vi "loadHTOutcount.vi"() -> ()   [LabVIEW 2012]
uses:
  <vilib>/Utility/file.llb/Read From Spreadsheet File (string).vi
panel:
  out "output cluster 2":T1
  in  "input cluster 2":T1
  out "before substring 5":string
  out "before substring 4":string
  in  "path":path=path "C:/temp/ht"
  out "filenames":string[](array[string])
  out "time stamp":timestamp
  out "SQLDateTime":string
  out "output cluster":T2
  in  "input cluster":T2
  out "all rows":string[][](array[string])
  out "size(s)":i32[](array[numeric])
  in  "file path (dialog if empty)":path=path "C:/temp/ht/G04N19.1S-1_09_07_00.txt"
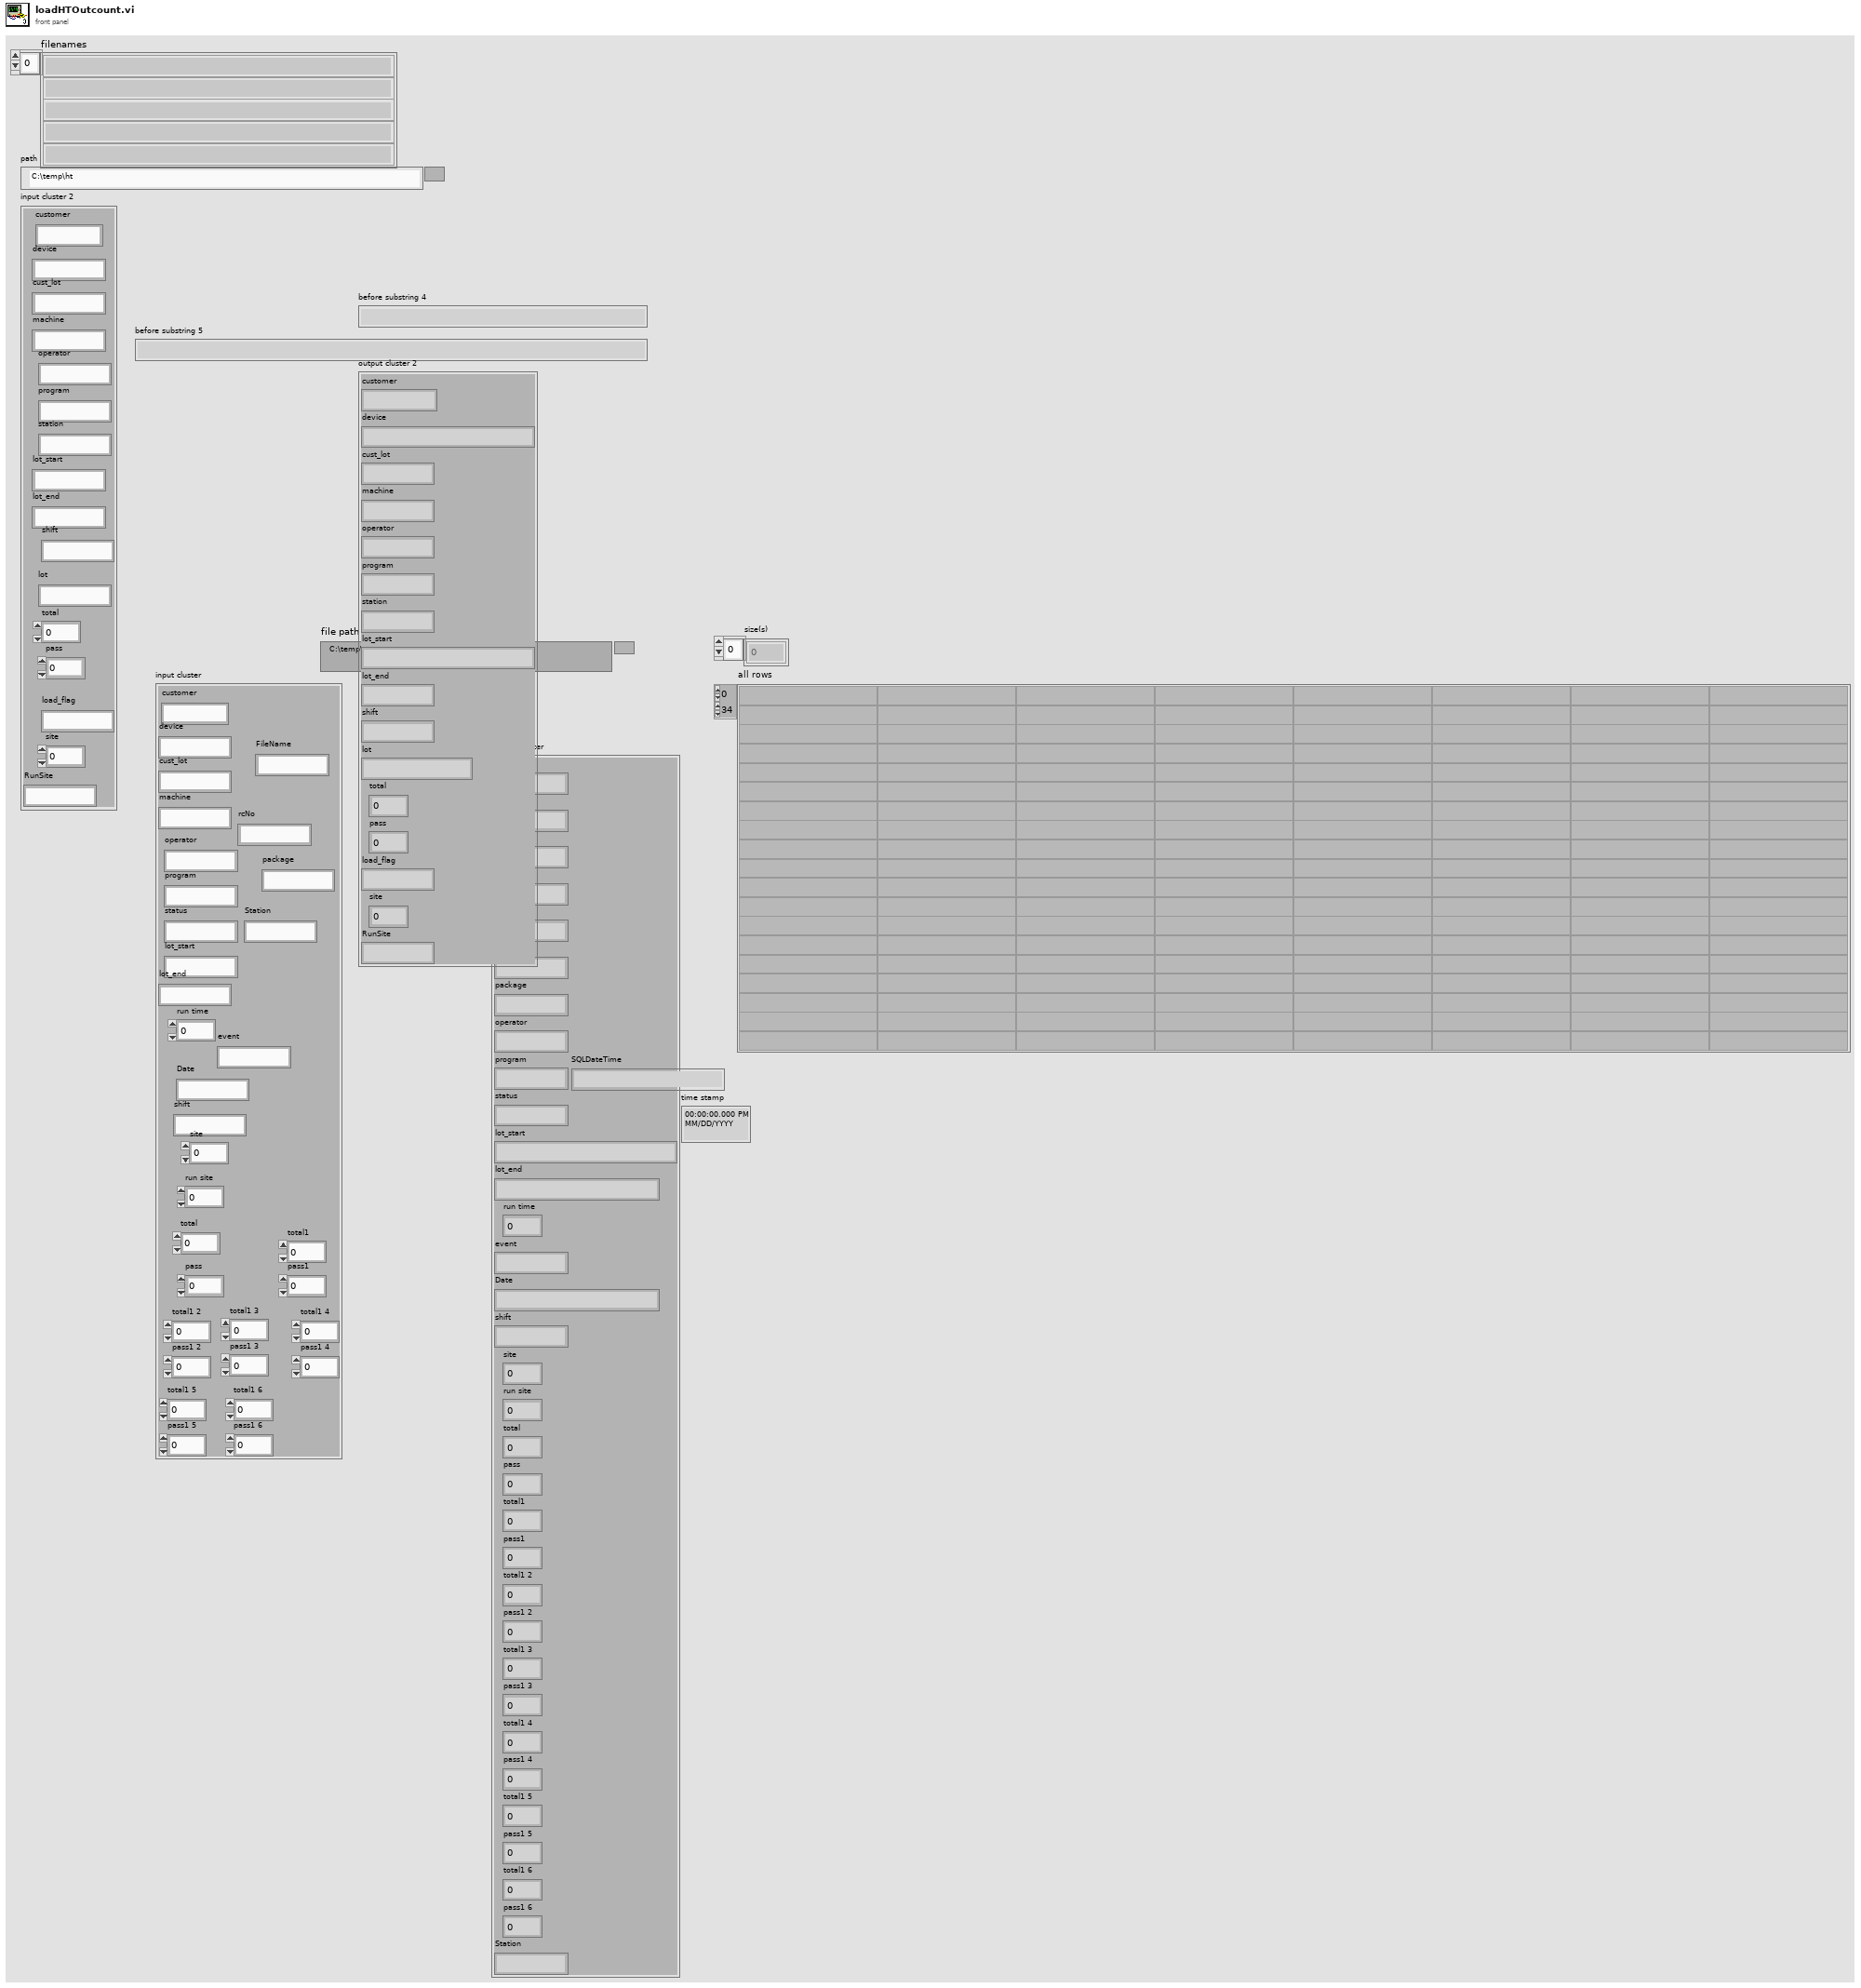
[diagram p1: front panel]
types:
  T1 = cluster{"customer":string, "device":string, "cust_lot":string, "machine":string, "operator":string, "program":string, "station":string, "lot_start":string, "lot_end":string, "shift":string, "lot":string, "total":dbl, "pass":dbl, "load_flag":string, "site":dbl, "RunSite":string}
  T2 = cluster{"customer":string, "device":string, "FileName":string, "cust_lot":string, "machine":string, "rcNo":string, "package":string, "operator":string, "program":string, "status":string, "lot_start":string, "lot_end":string, "run time":dbl, "event":string, "Date":string, "shift":string, "site":dbl, "run site ":dbl, "total":dbl, "pass":dbl, "total1":dbl, "pass1":dbl, "total1 2":dbl, "pass1 2":dbl, "total1 3":dbl, "pass1 3":dbl, "total1 4":dbl, "pass1 4":dbl, "total1 5":dbl, "pass1 5":dbl, "total1 6":dbl, "pass1 6":dbl, "Station":string}
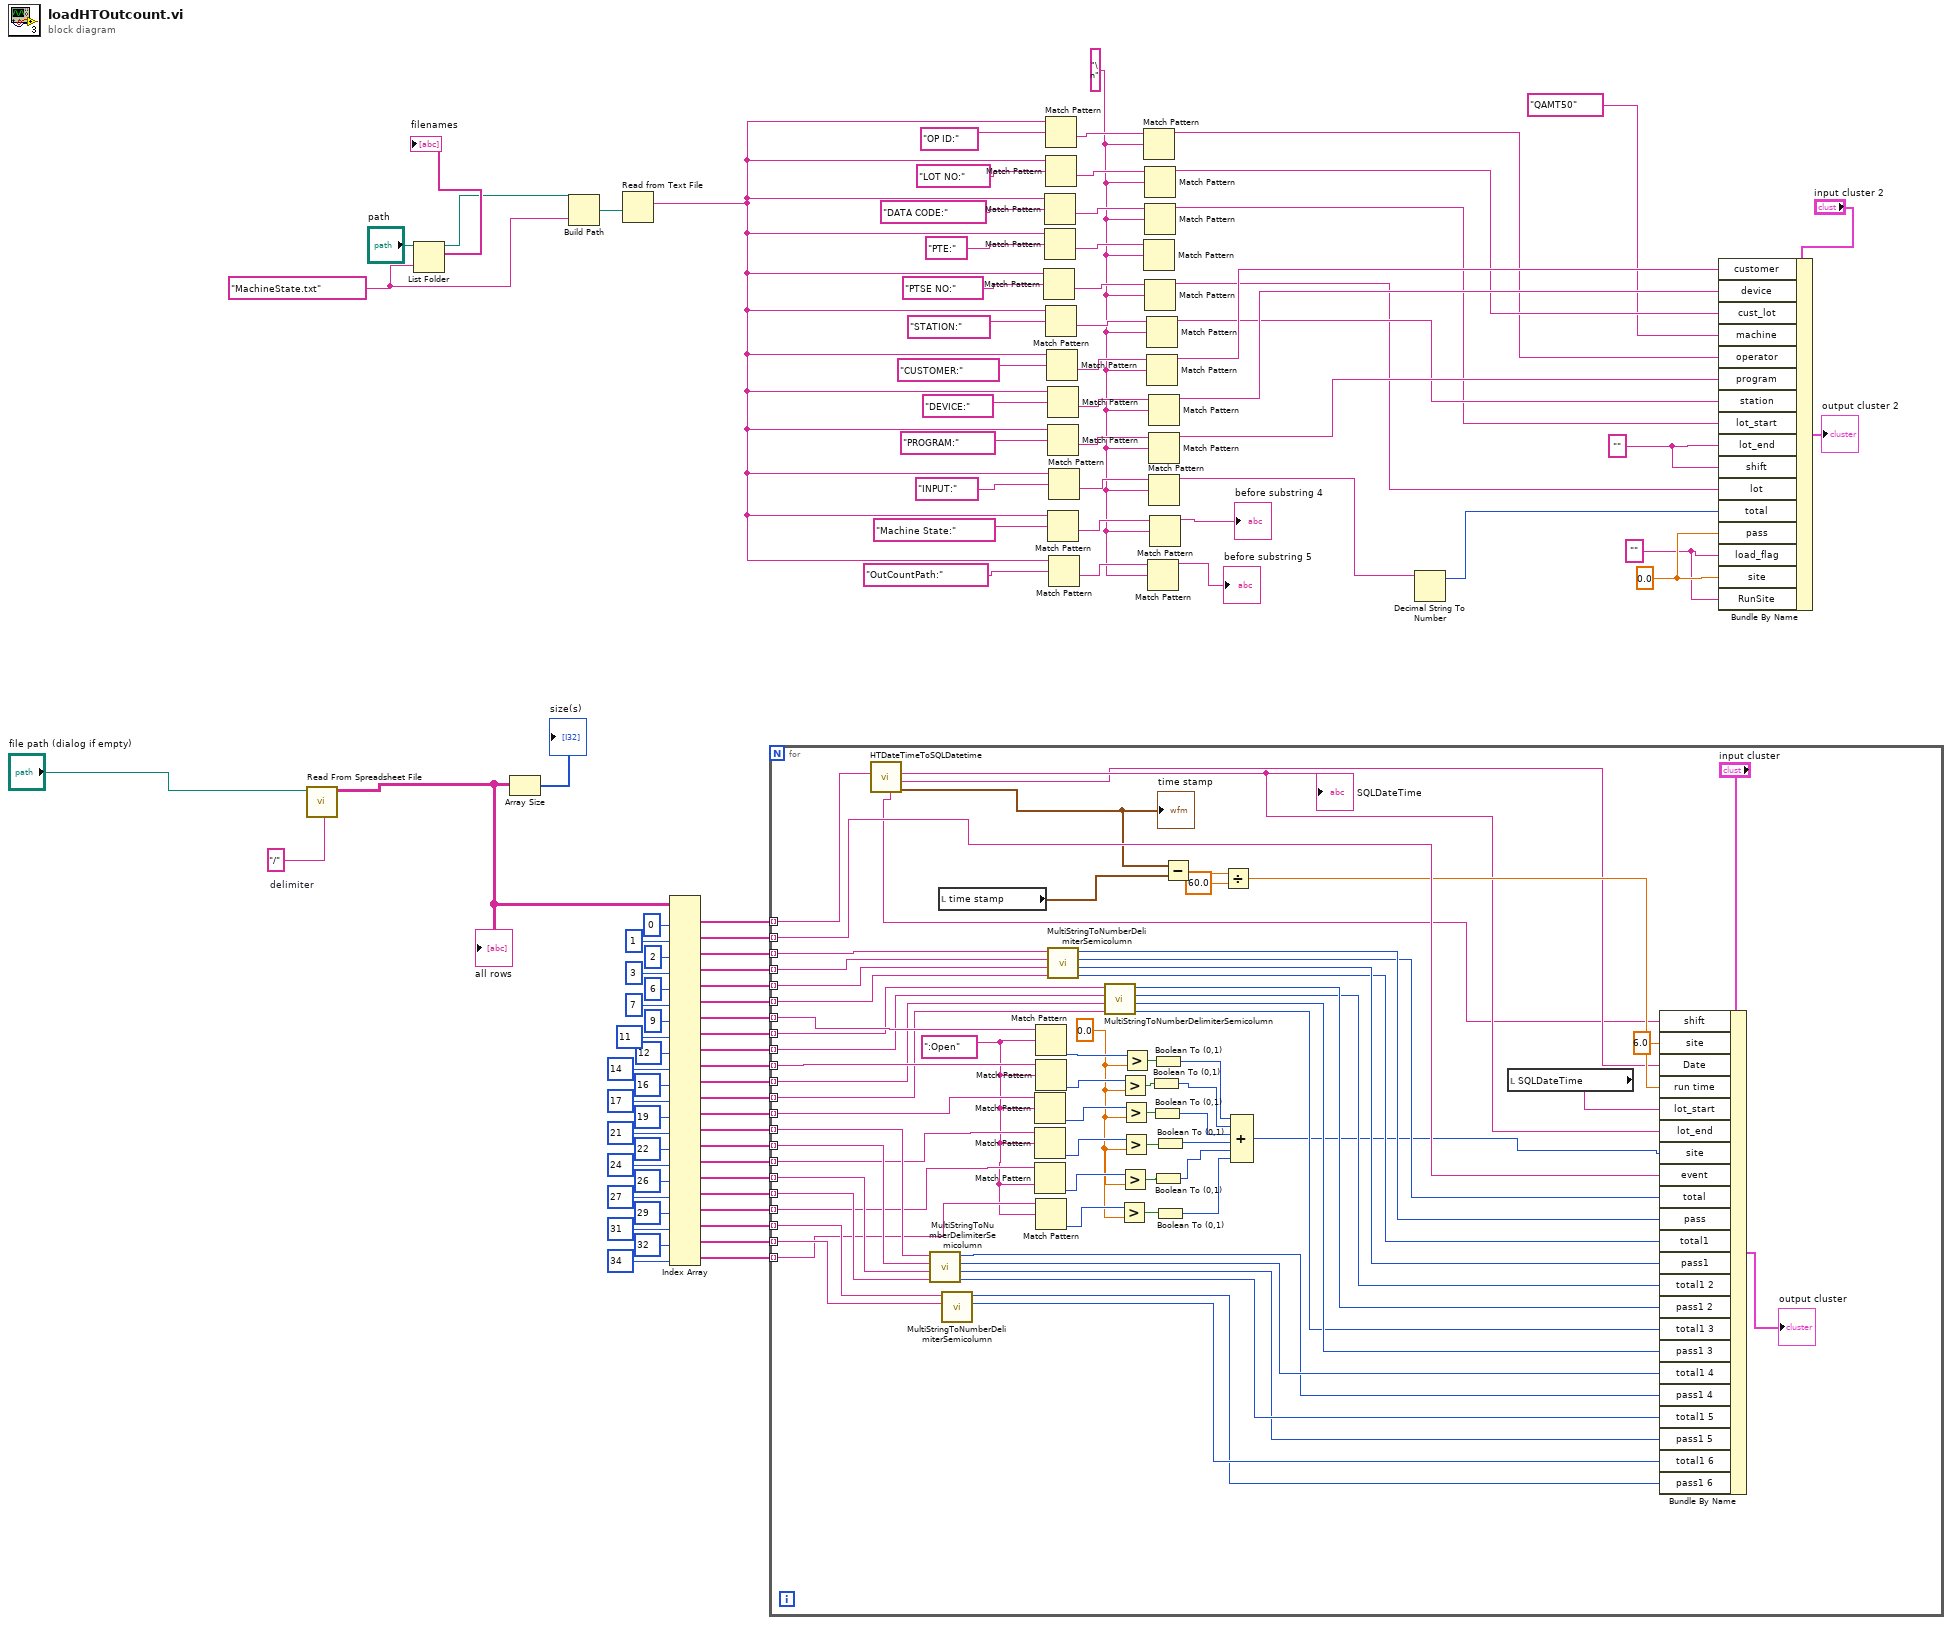
[diagram p0: block diagram]
diagram:
  w3 = "" ("load_flag")
  w4 = 0.0 ("site")
  w7 = "" ("lot_end")
  w1 = "\n" ("regular expression")
  w20 = "MachineState.txt" ("pattern")
  w97 = "/"  # delimiter
  n1 = call-poly <vilib>:"Read From Spreadsheet File.vi"("delimiter (\\t)"=w97, "file path (dialog if empty)"="file path (dialog if empty)") -> ("all rows"=w94:string[][])  [unwired: 5 in, 4 out]
  "all rows" <- w94
  n2 = List Folder(path="path", pattern=w20) -> (path out=w48:path, filenames=→"filenames":string[])  [unwired: 2 in, 2 out]
  n3 = Array Size(array=w94) -> (size(s)=→"size(s)":i32[])
  n4 = Build Path(base path=w48, name or relative path=w20) -> (appended path=w46:path)
  n5 = Read from Text File(file (use dialog)=w46) -> (text=w45:string)  [unwired: 3 in, 3 out]
  n6 = Index Array(array=w94, index (col) #1=0 ("disabled index (col)"), index (col) #2=1 ("index (col)"), index (col) #3=2 ("index (col)"), index (col) #4=3 ("index (col)"), index (col) #5=6 ("index (col)"), index (col) #6=7 ("index (col)"), index (col) #7=9 ("index (col)"), index (col) #8=11 ("index (col)"), index (col) #9=12 ("index (col)"), index (col) #10=14 ("index (col)"), index (col) #11=16 ("index (col)"), index (col) #12=17 ("index (col)"), index (col) #13=19 ("index (col)"), index (col) #14=21 ("index (col)"), index (col) #15=22 ("index (col)"), index (col) #16=24 ("index (col)"), index (col) #17=26 ("index (col)"), index (col) #18=27 ("index (col)"), index (col) #19=29 ("index (col)"), index (col) #20=31 ("index (col)"), index (col) #21=32 ("index (col)"), index (col) #22=34 ("index (col)")) -> (element #1=w92:string[], element #2=w90:string[], element #3=w87:string[], element #4=w86:string[], element #5=w83:string[], element #6=w82:string[], element #7=w80:string[], element #8=w77:string[], element #9=w76:string[], element #10=w74:string[], element #11=w71:string[], element #12=w70:string[], element #13=w68:string[], element #14=w65:string[], element #15=w64:string[], element #16=w62:string[], element #17=w59:string[], element #18=w58:string[], element #19=w56:string[], element #20=w53:string[], element #21=w52:string[], element #22=w50:string[])  [unwired: 22 in]
  n7 = for {
    tunnel: w92 -> [w166] mode=indexing
    tunnel: w90 -> [w130] mode=indexing
    tunnel: w87 -> [w164] mode=indexing
    tunnel: w86 -> [w163] mode=indexing
    tunnel: w83 -> [w162] mode=indexing
    tunnel: w82 -> [w161] mode=indexing
    tunnel: w80 -> [w165] mode=indexing
    tunnel: w77 -> [w160] mode=indexing
    tunnel: w76 -> [w159] mode=indexing
    tunnel: w74 -> [w158] mode=indexing
    tunnel: w71 -> [w157] mode=indexing
    tunnel: w70 -> [w156] mode=indexing
    tunnel: w68 -> [w155] mode=indexing
    tunnel: w65 -> [w154] mode=indexing
    tunnel: w64 -> [w153] mode=indexing
    tunnel: w62 -> [w152] mode=indexing
    tunnel: w59 -> [w151] mode=indexing
    tunnel: w58 -> [w150] mode=indexing
    tunnel: w56 -> [w149] mode=indexing
    tunnel: w53 -> [w148] mode=indexing
    tunnel: w52 -> [w147] mode=indexing
    tunnel: w50 -> [w129] mode=indexing
    w121 = 0.0 ("y")
    w128 = ":Open" ("regular expression")
    n8 = call "HTDateTimeToSQLDatetime.vi"("HTDateTime"=w166) -> ("time stamp"=w105:timestamp, "date string"=w100:string, "SQLDateTime"=w101:string, "Shift"=w98:string)  [unwired: 7 in]
    "SQLDateTime" <- w101
    "time stamp" <- w105
    n9 = call "MultiStringToNumberDelimiterSemicolumn.vi"("input string 4"=w150, "input string 3"=w151, "input string 2"=w153, "input string"=w154) -> ("number 4"=w143:i32, "number 3"=w142:i32, "number 2"=w141:i32, "number"=w140:i32)  [unwired: 4 in]
    n10 = local read "time stamp"() -> (w106:timestamp)
    n11 = call "MultiStringToNumberDelimiterSemicolumn.vi"("input string 2"=w147, "input string"=w148) -> ("number 2"=w145:i32, "number"=w144:i32)  [unwired: 6 in, 2 out]
    n12 = Match Pattern(string=w155, regular expression=w128) -> (offset past match=w125:i32)  [unwired: 1 in, 3 out]
    n13 = Match Pattern(string=w152, regular expression=w128) -> (offset past match=w124:i32)  [unwired: 1 in, 3 out]
    n14 = Match Pattern(string=w149, regular expression=w128) -> (offset past match=w123:i32)  [unwired: 1 in, 3 out]
    n15 = Match Pattern(string=w165, regular expression=w128) -> (offset past match=w127:i32)  [unwired: 1 in, 3 out]
    n16 = Match Pattern(string=w158, regular expression=w128) -> (offset past match=w126:i32)  [unwired: 1 in, 3 out]
    n17 = Match Pattern(string=w129, regular expression=w128) -> (offset past match=w122:i32)  [unwired: 1 in, 3 out]
    n18 = call "MultiStringToNumberDelimiterSemicolumn.vi"("input string 4"=w161, "input string 3"=w162, "input string 2"=w163, "input string"=w164) -> ("number 4"=w134:i32, "number 3"=w135:i32, "number 2"=w132:i32, "number"=w133:i32)  [unwired: 4 in]
    n19 = call "MultiStringToNumberDelimiterSemicolumn.vi"("input string 4"=w156, "input string 3"=w157, "input string 2"=w159, "input string"=w160) -> ("number 4"=w138:i32, "number 3"=w139:i32, "number 2"=w136:i32, "number"=w137:i32)  [unwired: 4 in]
    n20 = Greater?(x=w122, y=w121) -> (0:w117:bool)
    n21 = Greater?(x=w126, y=w121) -> (0:w119:bool)
    n22 = Greater?(x=w123, y=w121) -> (0:w115:bool)
    n23 = Greater?(x=w125, y=w121) -> (0:w116:bool)
    n24 = Greater?(x=w124, y=w121) -> (0:w118:bool)
    n25 = Greater?(x=w127, y=w121) -> (0:w120:bool)
    n26 = Boolean To (0,1)(Boolean=w119) -> (0, 1=w113:i16)
    n27 = Boolean To (0,1)(Boolean=w116) -> (0, 1=w112:i16)
    n28 = Boolean To (0,1)(Boolean=w120) -> (0, 1=w114:i16)
    n29 = Boolean To (0,1)(Boolean=w115) -> (0, 1=w110:i16)
    n30 = Boolean To (0,1)(Boolean=w118) -> (0, 1=w111:i16)
    n31 = Boolean To (0,1)(Boolean=w117) -> (0, 1=w109:i16)
    n32 = Subtract(x=w105, y=w106) -> (x-y=w104:dbl)
    n33 = Divide(x=w104, y=60.0) -> (x/y=w102:dbl)
    n34 = Compound Arithmetic op=ADD(w114, w113, w112, w111, w110, w109) -> (w108:i16)
    n35 = local read "SQLDateTime"() -> (w107:string)
    n36 = Bundle By Name(cluster="input cluster", "shift"=w98, "site"=6.0, "Date"=w100, "run time"=w102, "lot_start"=w107, "lot_end"=w101, "site"=w108, "event"=w130, "total"=w132, "pass"=w133, "total1"=w134, "pass1"=w135, "total1 2"=w136, "pass1 2"=w137, "total1 3"=w138, "pass1 3"=w139, "total1 4"=w141, "pass1 4"=w140, "total1 5"=w143, "pass1 5"=w142, "total1 6"=w145, "pass1 6"=w144) -> (→"output cluster":T2)
  }
  n37 = Match Pattern(string=w45, regular expression="PTSE NO:") -> (after substring=w35:string)  [unwired: 1 in, 3 out]
  n38 = Match Pattern(string=w45, regular expression="DATA CODE:") -> (after substring=w39:string)  [unwired: 1 in, 3 out]
  n39 = Match Pattern(string=w45, regular expression="PTE:") -> (after substring=w37:string)  [unwired: 1 in, 3 out]
  n40 = Match Pattern(string=w45, regular expression="OP ID:") -> (after substring=w43:string)  [unwired: 1 in, 3 out]
  n41 = Match Pattern(string=w45, regular expression="LOT NO:") -> (after substring=w41:string)  [unwired: 1 in, 3 out]
  n42 = Match Pattern(string=w45, regular expression="STATION:") -> (after substring=w22:string)  [unwired: 1 in, 3 out]
  n43 = Match Pattern(string=w45, regular expression="CUSTOMER:") -> (after substring=w33:string)  [unwired: 1 in, 3 out]
  n44 = Match Pattern(string=w45, regular expression="DEVICE:") -> (after substring=w31:string)  [unwired: 1 in, 3 out]
  n45 = Match Pattern(string=w45, regular expression="PROGRAM:") -> (after substring=w29:string)  [unwired: 1 in, 3 out]
  n46 = Match Pattern(string=w45, regular expression="Machine State:") -> (after substring=w25:string)  [unwired: 1 in, 3 out]
  n47 = Match Pattern(string=w45, regular expression="INPUT:") -> (after substring=w27:string)  [unwired: 1 in, 3 out]
  n48 = Match Pattern(string=w45, regular expression="OutCountPath:") -> (after substring=w23:string)  [unwired: 1 in, 3 out]
  n49 = Match Pattern(string=w43, regular expression=w1) -> (before substring=w13:string)  [unwired: 1 in, 3 out]
  n50 = Match Pattern(string=w37, regular expression=w1) -> ()  [unwired: 1 in, 4 out]
  n51 = Match Pattern(string=w41, regular expression=w1) -> (before substring=w14:string)  [unwired: 1 in, 3 out]
  n52 = Match Pattern(string=w39, regular expression=w1) -> (before substring=w8:string)  [unwired: 1 in, 3 out]
  n53 = Match Pattern(string=w35, regular expression=w1) -> (before substring=w10:string)  [unwired: 1 in, 3 out]
  n54 = Match Pattern(string=w22, regular expression=w1) -> (before substring=w11:string)  [unwired: 1 in, 3 out]
  n55 = Match Pattern(string=w33, regular expression=w1) -> (before substring=w16:string)  [unwired: 1 in, 3 out]
  n56 = Match Pattern(string=w23, regular expression=w1) -> (before substring=→"before substring 5":string)  [unwired: 1 in, 3 out]
  n57 = Match Pattern(string=w31, regular expression=w1) -> (before substring=w15:string)  [unwired: 1 in, 3 out]
  n58 = Match Pattern(string=w29, regular expression=w1) -> (before substring=w12:string)  [unwired: 1 in, 3 out]
  n59 = Match Pattern(string=w27, regular expression=w1) -> (before substring=w6:string)  [unwired: 1 in, 3 out]
  n60 = Match Pattern(string=w25, regular expression=w1) -> (before substring=→"before substring 4":string)  [unwired: 1 in, 3 out]
  n61 = Decimal String To Number(string=w6) -> (offset past number=w5:i32)  [unwired: 2 in, 1 out]
  n62 = Bundle By Name(cluster="input cluster 2", "customer"=w16, "device"=w15, "cust_lot"=w14, "machine"="QAMT50", "operator"=w13, "program"=w12, "station"=w11, "lot_start"=w8, "lot_end"=w7, "shift"=w7, "lot"=w10, "total"=w5, "pass"=w4, "load_flag"=w3, "site"=w4, "RunSite"=w3) -> (→"output cluster 2":T1)
